vi "Intro_2.vi"() -> ()   [LabVIEW 2010]
panel:
  out "x > y?":bool
  out "Limit Value(0-1) 2":dbl min=0.0 max=1.0
  in  "Limit Value(0-1)":dbl(knob) min=0.0 max=1.0 scale=0.0..1.0
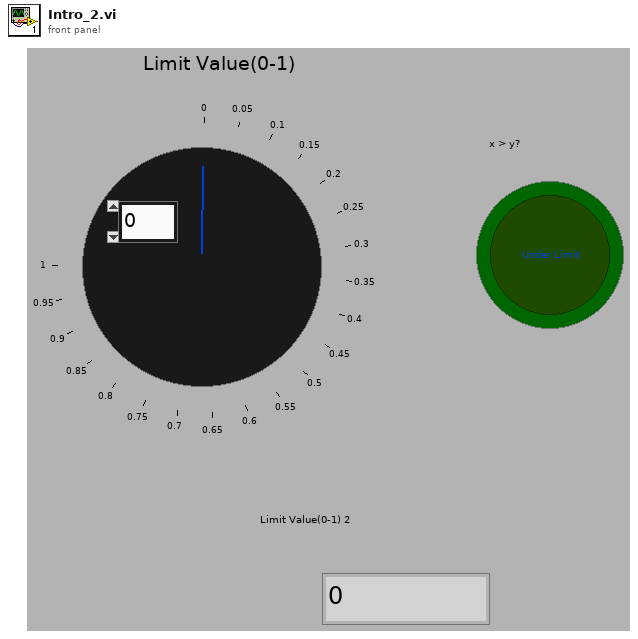
[diagram p1: front panel]
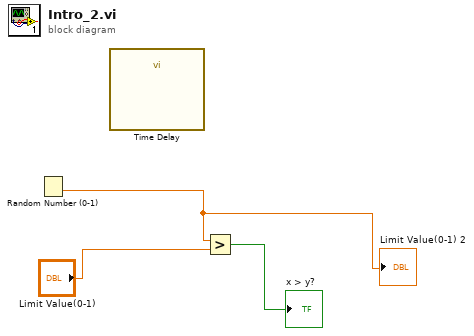
[diagram p0: block diagram]
diagram:
  n1 = Random Number (0-1)() -> (number: 0 to 1=w1:dbl)
  "Limit Value(0-1) 2" <- w1
  n2 = call "Time Delay"() -> ()  [unwired: 11 in, 1 out]
  n3 = Greater?(x=w1, y="Limit Value(0-1)") -> (0:→"x > y?":bool)
